vi "Subvi_Online_SVM_SWLDA_newMethod_in_분석기.vi"(0 "rate":dbl=500.0 caption="Rate" format="%0.2f", 1 "samples per channel":i32=25, 3 "in":T1, 4 "Group Number":i32, 5 "Brain_data_source":dbl[][](array[numeric]) caption="EEG_Raw_Data" format="%0.3f", 7 "Target_Flash_Order":i64[][](array[numeric]), 8 "Value":T1, 9 "svm_model_file":string, 11 "W":dbl[][](array[numeric]), 12 "Matrix":T1, 13 "전체_Selected":i32[](array[numeric]), 14 "Target":path, 15 "Selected":i32[](array[numeric]), 16 "Nontarget":path) -> (17 "EPR_발생_total":i16[](array[numeric]), 20 "output-0~8":i32, 21 "decision":dbl[](array[numeric]), 25 "SWLDA":dbl[](array[numeric]), 27 "ERP_Parameters":dbl[][](array[numeric]))   [LabVIEW 2014]
uses:
  <vilib>/Analysis/Matrix/Datatypes/RealMatrix.ctl
  <vilib>/Analysis/3filter.llb/Filter Passband Type.ctl
  <vilib>/Analysis/baseanly.llb/Mean (DBL).vi
  <vilib>/Analysis/3filter.llb/Butterworth Filter (DBL).vi
  <vilib>/Utility/file.llb/Read From Spreadsheet File (DBL).vi
  <vilib>/Analysis/Matrix/Numeric/Conversions/Array To Matrix - RA.vi
  <vilib>/Analysis/Matrix/Numeric/Multiply/Multiply - RM,RM.vi
  <vilib>/Analysis/Matrix/Numeric/Subtract/Subtract - RM,RM.vi
  <vilib>/Analysis/Matrix/Numeric/Conversions/Matrix To Array - RM.vi
  <vilib>/Analysis/NI_AALBase.lvlib
  <vilib>/Analysis/Matrix/NI_Matrix.lvlib
  <vilib>/Analysis/Matrix/Numeric/Conversions/Array To Matrix - RA2.vi
  <vilib>/gmath/NI_Gmath.lvlib
panel:
  out "size(s) 2":i32
  out "Real":dbl
  out "deleted portion":dbl[][](array[numeric])
  out "2-D Array of Real 3":dbl[][](array[numeric])
  out "2-D Array of Real 2":dbl[][](array[numeric])
  out "2-D Array of Real":dbl[][](array[numeric])
  out "1-D Array of Real":dbl[](array[numeric])
  out "SWLDA_original":dbl[][](array[numeric])
  out "size(s)":i32[](array[numeric])
  in  "LDA":path=path "C:/Users/Administrator/Desktop/공공복지안전사업연구-노수진/파일럿20130902/LDA_Matrix_Value.xls"
  out "전치된 배열":dbl[][](array[numeric])
  out "#channel":i32
  out "#sti 6":i32
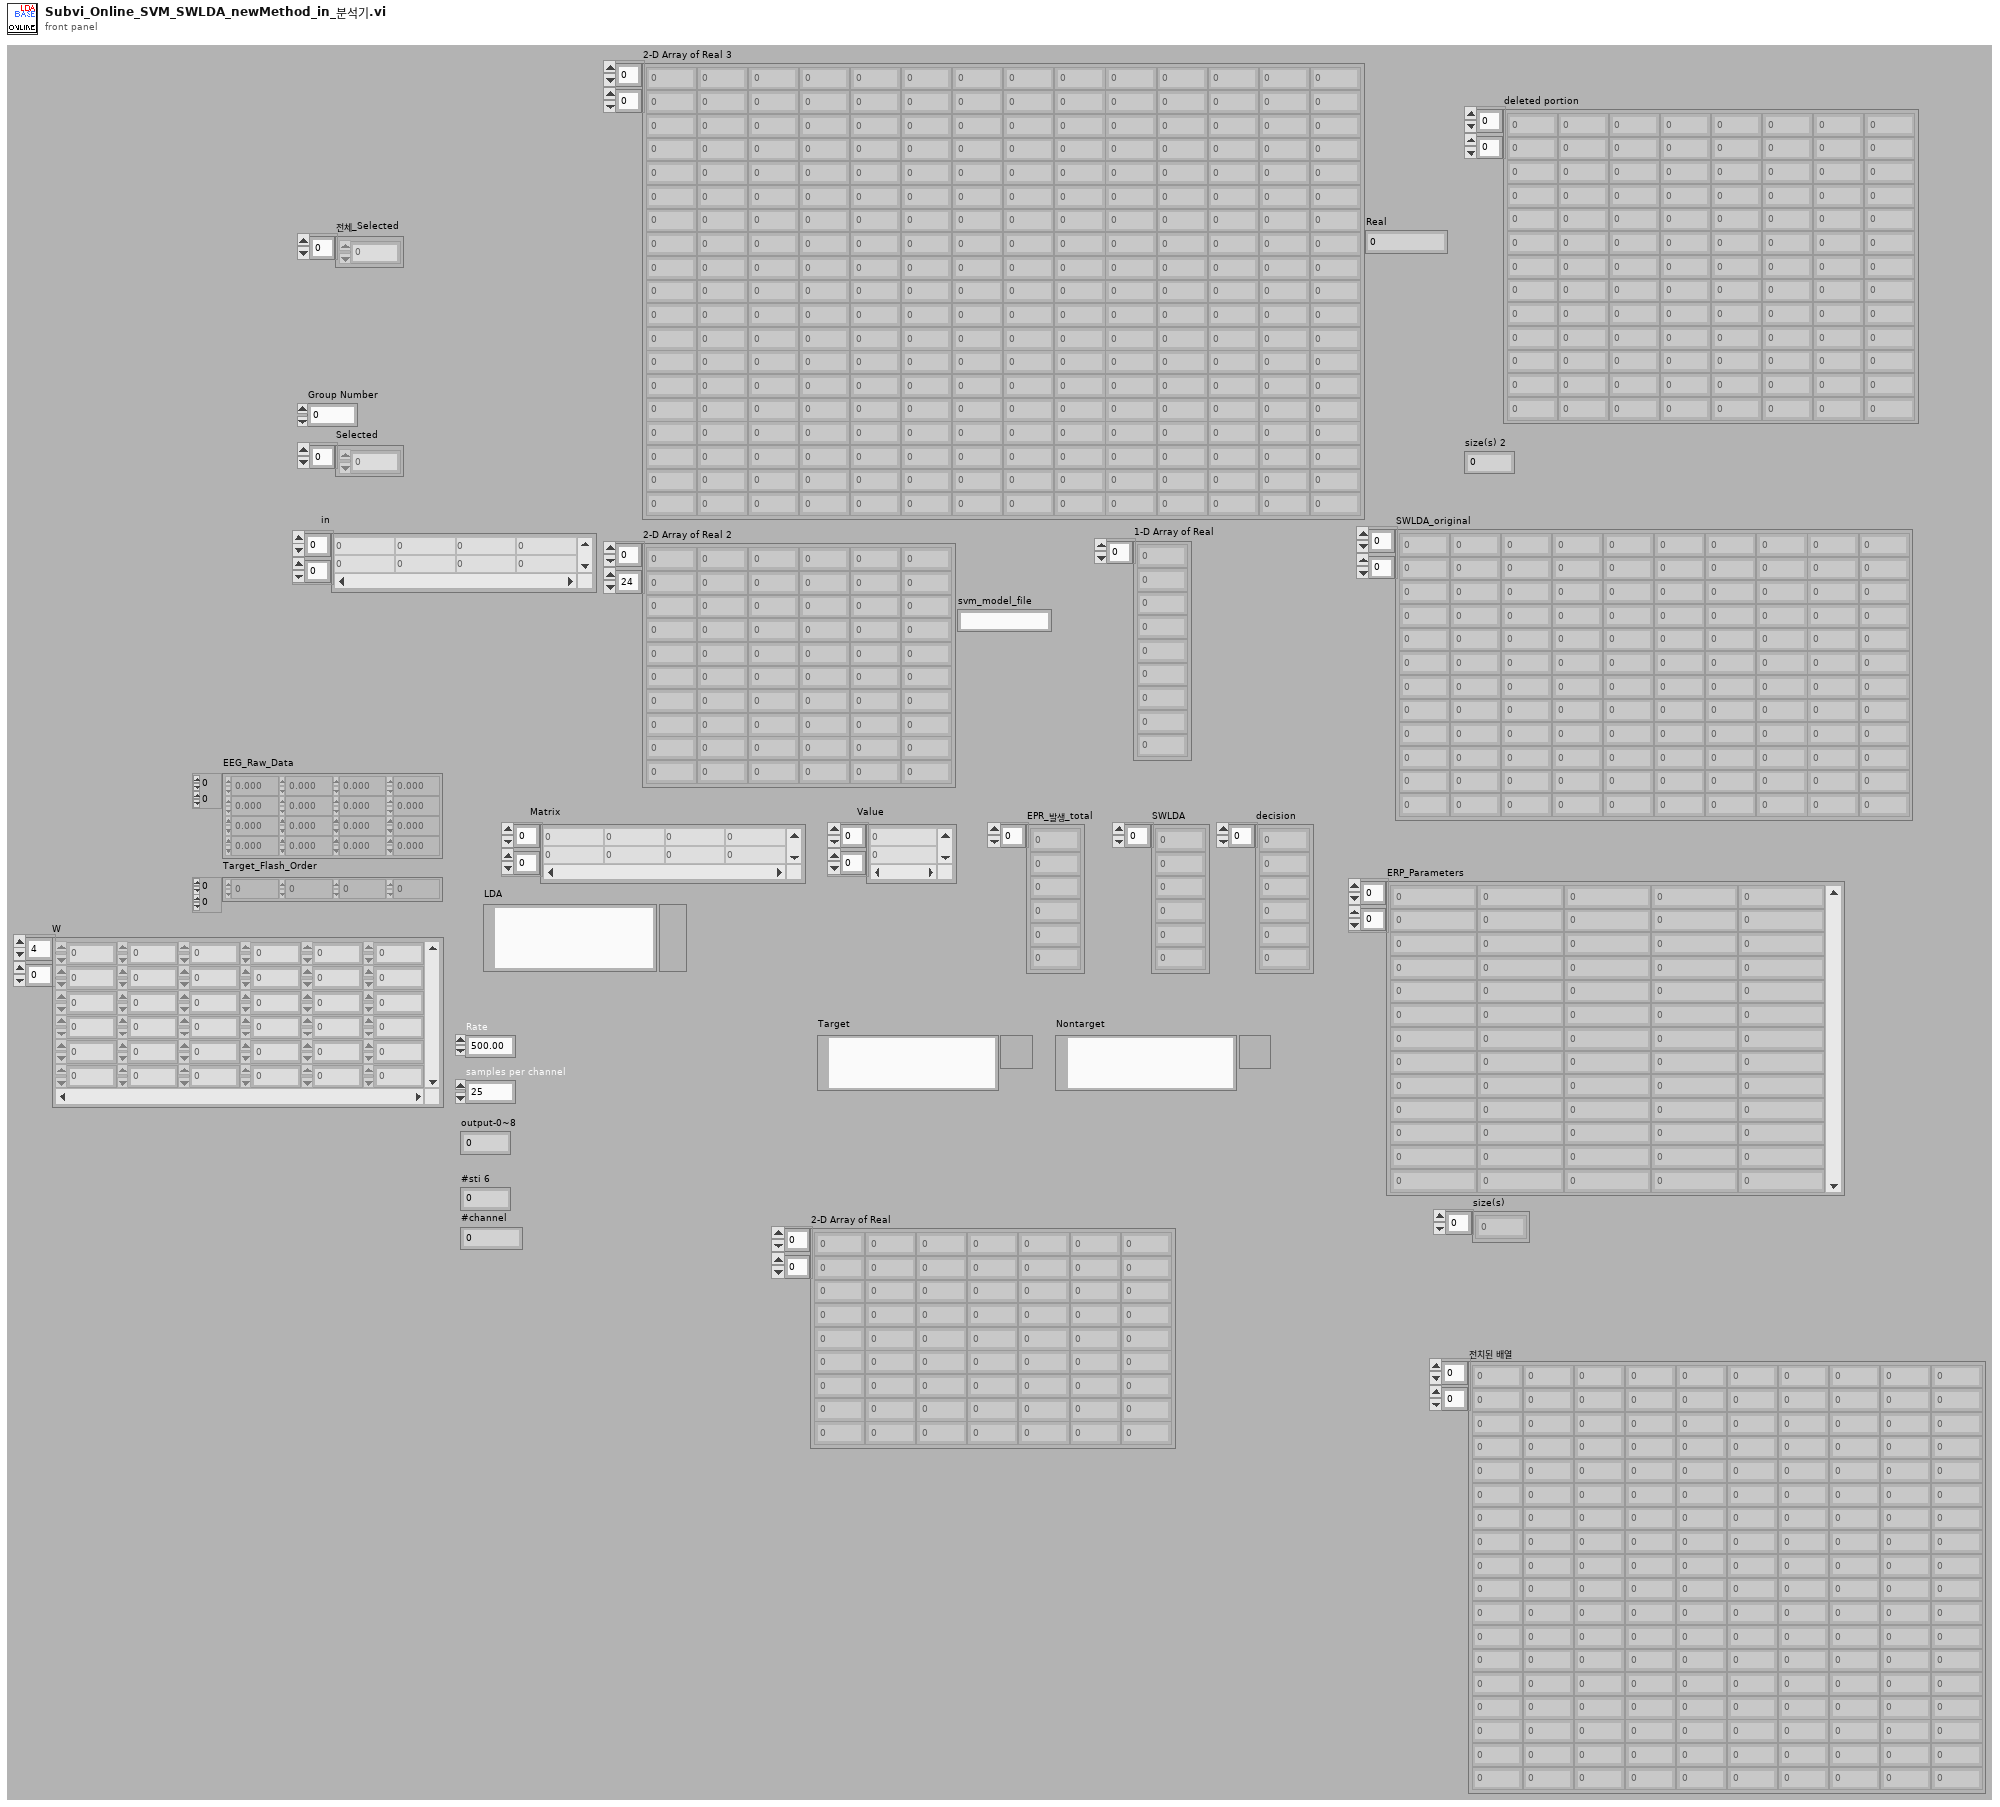
[diagram p1: front panel]
types:
  T1 = typedef "NI_Matrix.lvlib/RealMatrix.ctl" = dbl[][]
  T2 = typedef "NI_AALBase.lvlib/Filter Passband Type.ctl" = enum32{"Lowpass", "Highpass", "Bandpass", "Bandstop"}
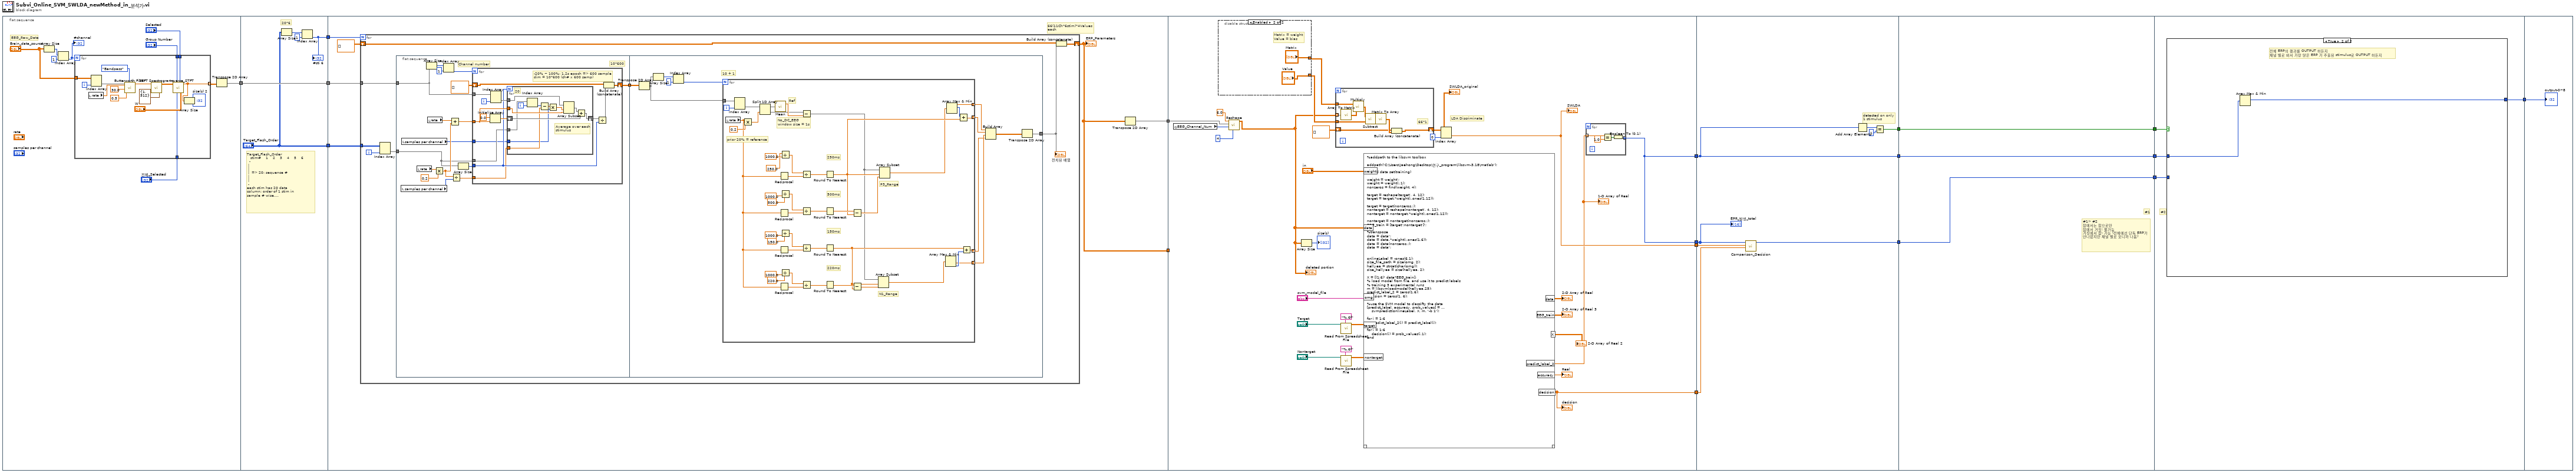
[diagram p0: block diagram]
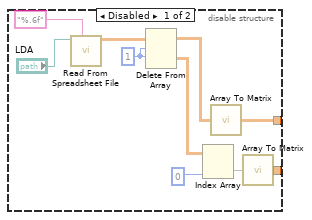
[diagram p2: hidden frame]
diagram:
  n1 = flat-sequence {
    tunnel: [w22] -> w17
    tunnel: [w47] -> w16
    tunnel: ["Target_Flash_Order"] -> w15
    tunnel: w17 -> [w47]
    tunnel: [w44] -> w14
    tunnel: w16 -> [w53]
    tunnel: w15 -> [w52]
    tunnel: w14 -> [w51]
    tunnel: [w48] -> w13
    tunnel: [w49] -> w12
    tunnel: w13 -> [w168]
    tunnel: w12 -> [_]
    tunnel: [w182] -> w11
    tunnel: [w182] -> w9
    tunnel: [w179] -> w7
    tunnel: [w163] -> w3
    tunnel: w11 -> [w215]
    tunnel: [w216] -> w10
    tunnel: w9 -> [w214]
    tunnel: w7 -> [w213]
    tunnel: [w215] -> w6
    tunnel: w3 -> [w212]
    tunnel: [w211] -> w2
    tunnel: w10 -> [w220]
    tunnel: w6 -> [w221]
    tunnel: [w221] -> w5
    tunnel: [w220] -> w4
    tunnel: w2 -> [w219]
    tunnel: [w219] -> w1
    tunnel: [w225] -> w8
    tunnel: w5 -> [w223]
    tunnel: w4 -> [w224]
    tunnel: w1 -> [w222]
    tunnel: w8 -> [w229]
    frame #0 {
      # "EEG_Raw_Data"
      n2 = Array Size(array="Brain_data_source") -> (size(s)=w23:i32[])
      n3 = Index Array(array=w23, index=1) -> (element=w25:i32)
      "#channel" <- w25
      n4 = for {
        N: w25 -> [_]
        tunnel: "Brain_data_source" -> [w42]
        tunnel: [w28] -> w26 mode=indexing
        tunnel: "Selected" -> [w31]
        tunnel: "Group Number" -> [w30]
        tunnel: "전체_Selected" -> [w29]
        i -> [w41]
        n5 = local read "rate"() -> (w36:dbl)
        n6 = Index Array(array=w42, index (col)=w41) -> (element=w40:dbl[])  [unwired: 1 in]
        n7 = call-poly <vilib>:"Butterworth Filter.vi"("filter type"=Filter_Passband_Type."Bandpass", "low cutoff freq: fl"=0.5, "high cutoff freq: fh"=30.0, "sampling freq: fs"=w36, "X"=w40) -> ("Filtered X"=w33:dbl[])  [unwired: 3 in, 1 out]
        n8 = call <vilib>:"STFT Spectrograms.vi"("time-freq sampling info"=cluster{"time steps":i32, "frequency bins":i32} {"time steps"=1, "frequency bins"=512}, "X"=w33) -> ("STFT Spectrogram {X}"=w34:dbl[][])  [unwired: 8 in, 1 out]
        n9 = call "Inverse_STFT.vi"("Selected"=w31, "전체_Selected"=w29, "Group Number"=w30, "W"="W", "STFT Spectrogram {X}"=w34) -> ("Inverse_STFT"=w28:dbl[])  [unwired: 6 in]
        n10 = Array Size(array=w28) -> (size(s)=→"size(s) 2":i32)
      }
      n11 = Transpose 2D Array(2D array=w26) -> (transposed array=w22:dbl[][])
    }
    frame #1 {
      # "Target_Flash_Order\n   stim#    1    2    3    4    5    6    \n  -\n |\n |\n |  => 20: sequence # \n |\n |\n -\neach stim has 20 data\ncolumn: order of 1 stim in \nsample # wise...."
      # "20*6"
      n12 = Array Size(array="Target_Flash_Order") -> (size(s)=w46:i32[])
      n13 = Index Array(array=w46, index=1 ("인덱스")) -> (element=w44:i32)
      "#sti 6" <- w44
    }
    frame #2 {
      # "66(11Ch*6stim)*4Values\neach"
      n14 = for {
        N: w51 -> [_]
        tunnel: w53 -> [w60]
        tunnel: w52 -> [w59]
        shift-right: [w56] -> w49
        shift-left: dbl[][] [] -> [w55]
        i -> [w58]
        n15 = Index Array(array=w59, index (col)=w58) -> (element=w57:i64[])  [unwired: 1 in]
        n16 = flat-sequence {
          tunnel: w60 -> [w64]
          tunnel: w57 -> [w63]
          tunnel: [w62] -> w61
          tunnel: w61 -> [w108]
          tunnel: [w104] -> w54
          frame #0 {
            # "10*600"
            # "Channel number"
            n17 = local read "samples per channel"() -> (w71:i32)
            n18 = local read "samples per channel"() -> (w70:i32)
            n19 = local read "rate"() -> (w73:dbl)
            n20 = Array Size(array=w64) -> (size(s)=w67:i32[])
            n21 = local read "rate"() -> (w75:dbl)
            n22 = Multiply(x=w73, y=0.2) -> (x*y=w77:dbl)
            n23 = Index Array(array=w67, index=1) -> (element=w69:i32)
            n24 = Add(x=w75, y=w77) -> (x+y=w76:dbl)
            n25 = Divide(x=w77, y=w71) -> (x/y=w74:dbl)
            n26 = Array Size(array=w63) -> (size(s)=w66:i32)
            n27 = for {
              N: w69 -> [_]
              tunnel: w70 -> [w78]
              tunnel: w76 -> [w89]
              shift-right: [w82] -> w62
              shift-left: dbl[][] [] -> [w84]
              tunnel: w66 -> [w83]
              tunnel: w64 -> [w81]
              tunnel: w63 -> [w80]
              tunnel: w74 -> [w79]
              i -> [w91]
              # "-20% ~ 100%: 1.2s epoch => 600 sample\ndim = 10*600 (ch# x 600 samp)"
              n28 = Initialize Array(0.0 ("element"), w89) -> (w88:dbl[])
              n29 = Index Array(array=w81, index (col)=w91) -> (element=w90:dbl[])  [unwired: 1 in]
              n30 = for {
                N: w83 -> [_]
                tunnel: w90 -> [w103]
                shift-right: [w100] -> w86
                shift-left: w88 -> [w101]
                tunnel: w89 -> [w99]
                tunnel: w80 -> [w97]
                tunnel: w79 -> [w95]
                tunnel: w78 -> [w93]
                i -> [w98]
                # "Average over each\nstimulus"
                # "20"
                n31 = Index Array(array=w97, index=w98) -> (element=w96:i64)
                n32 = Subtract(x=w96, y=w95) -> (x-y=w94:dbl)
                n33 = Multiply(x=w94, y=w93) -> (x*y=w92:dbl)
                n34 = Array Subset(array=w103, index=w92, length=w99) -> (w102:dbl[])
                n35 = Add(x=w102, y=w101) -> (x+y=w100:dbl[])
              }
              n36 = Divide(x=w86, y=w83) -> (x/y=w85:dbl[])
              n37 = Build Array (concatenate)(w84, w85) -> (w82:dbl[][])
            }
          }
          frame #1 {
            # "10 + 1"
            n38 = Transpose 2D Array(2D array=w108) -> (transposed array=w106:dbl[][])
            n39 = Array Size(array=w106) -> (size(s)=w109:i32[])
            n40 = Index Array(array=w109, index=1) -> (element=w105:i32)
            n41 = for {
              N: w105 -> [_]
              tunnel: w106 -> [w158]
              tunnel: [w153] -> w113 mode=indexing
              tunnel: [w151] -> w112 mode=indexing
              tunnel: [w122] -> w111 mode=indexing
              tunnel: [w148] -> w110 mode=indexing
              i -> [w147]
              # "P3_Range"
              # "N1_Range"
              # "220ms"
              # "150ms"
              # "500ms"
              # "250ms"
              # "No_DC_EEG\nwindow size = 1s"
              # "Ref"
              # "prior 20% = reference"
              n42 = local read "rate"() -> (w129:dbl)
              n43 = Index Array(array=w158, index (col)=w147) -> (element=w150:dbl[])  [unwired: 1 in]
              n44 = Multiply(x=w129, y=0.2) -> (x*y=w156:dbl)
              n45 = Split 1D Array(array=w150, index=w156) -> (first subarray=w155:dbl[], second subarray=w146:dbl[])
              n46 = call-poly <vilib>:"Mean.vi"("X"=w155) -> ("mean"=w154:dbl)  [unwired: 1 out]
              n47 = Reciprocal(x=w129) -> (1/x=w145:dbl)
              n48 = Reciprocal(x=w129) -> (1/x=w144:dbl)
              n49 = Reciprocal(x=w129) -> (1/x=w143:dbl)
              n50 = Reciprocal(x=w129) -> (1/x=w142:dbl)
              n51 = Divide(x=250.0, y=1000.0) -> (x/y=w141:dbl)
              n52 = Divide(x=500.0, y=1000.0) -> (x/y=w140:dbl)
              n53 = Divide(x=150.0, y=1000.0) -> (x/y=w139:dbl)
              n54 = Divide(x=220.0, y=1000.0) -> (x/y=w138:dbl)
              n55 = Subtract(x=w146, y=w154) -> (x-y=w115:dbl[])
              n56 = Divide(x=w141, y=w145) -> (x/y=w128:dbl)
              n57 = Divide(x=w140, y=w144) -> (x/y=w127:dbl)
              n58 = Divide(x=w139, y=w143) -> (x/y=w126:dbl)
              n59 = Divide(x=w138, y=w142) -> (x/y=w125:dbl)
              n60 = Round To Nearest(number=w128) -> (nearest integer value=w118:dbl)
              n61 = Round To Nearest(number=w127) -> (nearest integer value=w124:dbl)
              n62 = Round To Nearest(number=w126) -> (nearest integer value=w120:dbl)
              n63 = Round To Nearest(number=w125) -> (nearest integer value=w123:dbl)
              n64 = Subtract(x=w124, y=w118) -> (x-y=w119:dbl)
              n65 = Subtract(x=w123, y=w120) -> (x-y=w121:dbl)
              n66 = Array Subset(array=w115, index=w120, length=w121) -> (w116:dbl[])
              n67 = Array Subset(array=w115, index=w118, length=w119) -> (w117:dbl[])
              n68 = Array Max & Min(array=w116) -> (min value=w122:dbl, min index (indices)=w149:i32)  [unwired: 2 out]
              n69 = Array Max & Min(array=w117) -> (max value=w153:dbl, max index (indices)=w152:i32)  [unwired: 2 out]
              n70 = Add(x=w152, y=w118) -> (x+y=w151:dbl)
              n71 = Add(x=w120, y=w149) -> (x+y=w148:dbl)
            }
            n72 = Build Array(w113, w112, w111, w110) -> (w107:dbl[][])
            n73 = Transpose 2D Array(2D array=w107) -> (transposed array=w104:dbl[][])
          }
        }
        n74 = Build Array (concatenate)(w55, w54) -> (w56:dbl[][])
        "전치된 배열" <- w54
      }
      "ERP_Parameters" <- w49
      n75 = Transpose 2D Array(2D array=w49) -> (transposed array=w48:dbl[][])
    }
    frame #3 {
      # "LDA Discriminate"
      # "66*1"
      n76 = global read "Control_Panel_정리.vi" "EEG_Channel_Num"() -> (w167:i32)
      n77 = disable-structure shown="Enabled" {
        disable-tunnel: [w190 "Matrix"] -> w180
        disable-tunnel: [w189 "Value"] -> w181
        frame Disabled {
          w192 = 1 ("인덱스 (행)")
          n78 = call-poly <vilib>:"Read From Spreadsheet File.vi"("format (%.3f)"="%.6f", "file path (dialog if empty)"="LDA") -> ("all rows"=w186:dbl[][])  [unwired: 5 in, 4 out]
          n79 = Delete From Array(array=w186, length=w192, index (row)=w192) -> (deleted portion=w195:dbl[][], array with subset deleted=w194:dbl[][])  [unwired: 1 in]
          n80 = Index Array(array=w195, index (col)=0 ("인덱스")) -> (element=w193:dbl[])  [unwired: 1 in]
          n81 = call-poly <vilib>:"Array To Matrix.vi"("Real 2D Array"=w194) -> ("Real Matrix"=w190:T1)
          n82 = call-poly <vilib>:"Array To Matrix.vi"("Real 1D Array"=w193) -> ("Real Matrix (Column Vector)"=w189:T1)
        }
        frame Enabled {
          # "Matrix = weight\nValue = bias"
        }
      }
      n83 = call "Reshape.vi"("Numeric"=4, "EEG_Channel_Num"=w167, "all rows"=w168, "Numeric 2"=6.0) -> ("Array"=w164:dbl[][])  [unwired: 7 in]
      "deleted portion" <- w164
      n84 = Array Size(array=w164) -> (size(s)=→"size(s)":i32[])
      n85 = for {
        tunnel: w180 -> [w202]
        tunnel: w181 -> [w208]
        shift-right: [w205] -> w183
        shift-left: dbl[][] [] -> [w204]
        tunnel: w164 -> [w203] mode=indexing
        n86 = call-poly <vilib>:"Array To Matrix.vi"("Real 1D Array"=w203) -> ("Real Matrix (Column Vector)"=w207:T1)
        n87 = call-poly <vilib>:"Multiply.vi"("Real Matrix B"=w207, "Real Matrix A"=w202) -> ("A * B"=w210:T1)
        n88 = call-poly <vilib>:"Subtract.vi"("Real Matrix B"=w208, "Real Matrix A"=w210) -> ("A - B"=w209:T1)
        n89 = call-poly <vilib>:"Matrix To Array.vi"("Real Matrix"=w209) -> ("Real 2D Array"=w206:dbl[][])
        n90 = Build Array (concatenate)(w204, w206) -> (w205:dbl[][])
      }
      "SWLDA_original" <- w183
      n91 = call-poly <vilib>:"Read From Spreadsheet File.vi"("format (%.3f)"="%.6f", "file path (dialog if empty)"="Target") -> ("all rows"=w176:dbl[][])  [unwired: 5 in, 4 out]
      n92 = call-poly <vilib>:"Read From Spreadsheet File.vi"("format (%.3f)"="%.6f", "file path (dialog if empty)"="Nontarget") -> ("all rows"=w175:dbl[][])  [unwired: 5 in, 4 out]
      n93 = script code="%addpath to the libsvm toolbox\n\naddpath('C:\\Users\\Jaehong\\Desktop\\연구_program\\libsvm-3.18\\matlab');\n\n%read data set(training)\n\nweight = weight';\nweight = weight(:,1);\nnonzeros = find(weight, 4);\n\ntarget = reshape(target', 4, 12);\ntarget = target.*weight(:,ones(1,12));\n\ntarget = target(nonzeros,:);\nnontarget = reshape(nontarget', 4, 12);\nnontarget = nontarget.*weight(:,ones(1,12));\n\nnontarget = nontarget(nonzeros,:);\nEEG_train = [target';nontarget']';\n\n%transpose\ndata = data';\ndata = data.*weight(:,ones(1,6));\ndata = data(nonzeros,:);\ndata = data';\n\n\nonlineLabel = -ones(6,1);\nsize_file_path = size(omg, 2);\nhellyea = strcat(char(omg));\nsize_hellyea = size(hellyea, 2);\n\nX = [(1:6)' data*EEG_train];\n% load model from file, and use it to predict labels\n% training 3 experimental runs\nm = libsvmloadmodel(hellyea,25);\npredict_label_2 = zeros(1,6);\ndecision = zeros(1, 6);\n\n%use the SVM model to classifty the data\n[predict_label, accuracy, prob_values] = ...\n    svmpredict(onlineLabel, X, m, '-b 1');\n\nfor i = 1:6\n    predict_label_2(i) = predict_label(i);\nend\nfor i = 1:6\n    decision(i) = prob_values(i,1);\nend"("weight"="in", "target"=w176, "nontarget"=w175, "data"=w164, "omg"="svm_model_file") -> ("predict_label_2"=w174:dbl[], "data"=→"2-D Array of Real":dbl[][], "EEG_train"=→"2-D Array of Real 3":dbl[][], "X"=→"2-D Array of Real 2":dbl[][], "accuracy"=→"Real":dbl, "decision"=w163:dbl[])  [unwired: 1 in, 1 out]
      "1-D Array of Real" <- w174
      "decision" <- w163
      n94 = Index Array(array=w183, index (col)=0 ("비활성화된 인덱스 (열)")) -> (element=w179:dbl[])  [unwired: 1 in]
      "SWLDA" <- w179
      n95 = for {
        tunnel: w174 -> [w201] mode=indexing
        tunnel: [w200] -> w182 mode=indexing
        n96 = Equal?(x=w201, y=1.0) -> (x = y?=w198:bool)
        n97 = Boolean To (0,1)(Boolean=w198) -> (0, 1=w200:i16)
      }
    }
    frame #4 {
      # "detected on only\n1 stimulus"
      n98 = call "Comparison_Decision.vi"("decision"=w212, "SWLDA"=w213, "EPR_발생_total"=w214) -> ("selected"=w211:i32)  [unwired: 8 in]
      n99 = Add Array Elements(numeric array=w215) -> (sum=w218:i16)
      n100 = Equal?(x=w218, y=i16 1) -> (x = y?=w216:bool)
      "EPR_발생_total" <- w214
    }
    frame #5 {
      # "#1> #2\n참에서는 참으로만\n참에서 거짓: 불가능\n거짓에서 참: 가능 (전체에선 단독 ERP가 안나왔지만 채널 별로 보니까 나옴)"
      # "#1"
    }
    frame #6 {
      # "#2"
      n101 = case shown="True" w224 {
        tunnel: [w226 w228] -> w225
        tunnel: w223 -> [_ w227]
        tunnel: w222 -> [w226 _]
        frame False {
        }
        frame True {
          # "전체 ERP의 결과를 OUTPUT 하든지\n채널 별로 봐서 가장 많은 ERP 가 추출된 stimulus로 OUTPUT 하든지"
          n102 = Array Max & Min(array=w227) -> (max index (indices)=w228:i32)  [unwired: 3 out]
        }
      }
    }
    frame #7 {
      "output-0~8" <- w229
    }
  }
